vi "Write String.vi"(8 "error in (no error)":errorcluster, 10 "String":string, 11 "Init in":refnum<class "Initialize.lvclass">) -> (0 "error out":errorcluster, 3 "Init out":refnum<class "Initialize.lvclass">)   [LabVIEW 2018, in "Initialize.lvclass"]
doc: "Initialize.lvclass:Write String.vi\n\nThis is the template for the Write String VI for the Initialize class.\n\nInstrument Communication Module Version 1.0\nOctober, 2020 Original Code Consulting Davita Bird\n www.originalcode.com"
uses:
  Initialize.lvclass
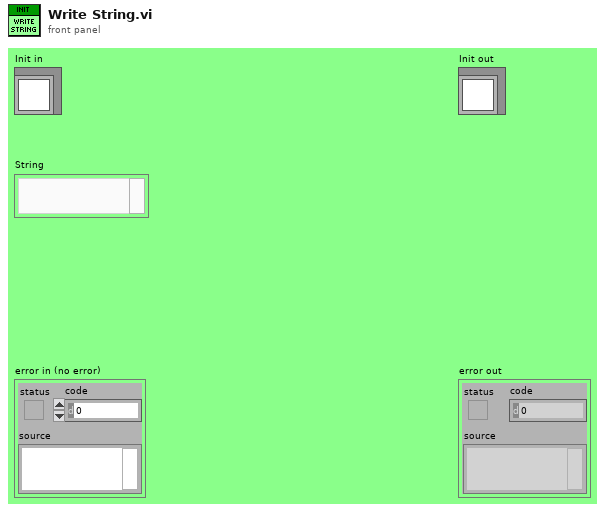
[diagram p1: front panel]
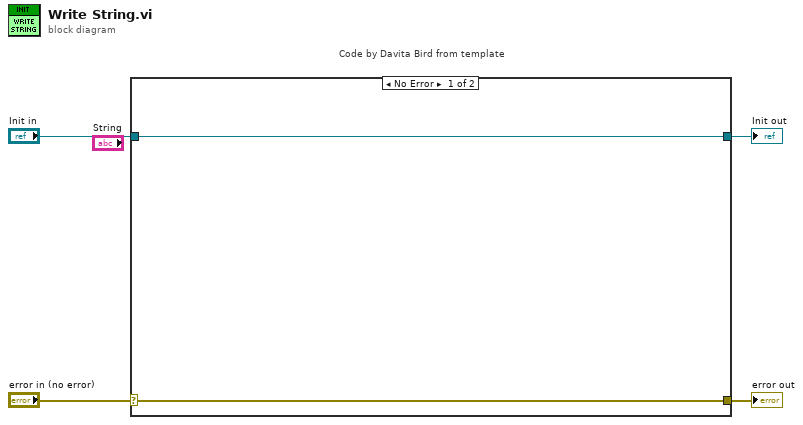
[diagram p0: block diagram]
diagram:
  n1 = case "Code by Davita Bird from template" shown="No Error" "error in (no error)" {
    selector: "error in (no error)" -> [w5 w8]
    tunnel: [w5 w8] -> w3
    tunnel: [w6 w7] -> w1
    tunnel: "Init in" -> [w6 w7]
    frame No Error {
    }
    frame Error {
    }
  }
  "error out" <- w3
  "Init out" <- w1
